vi "Read Calib File.vi"(8 "Inst type":T1=enum."Pressure Transducer", 11 "Calib File":path) -> (0 "Coefficients Found?":bool, 3 "Calib Constants":dbl[](array[numeric]))   [LabVIEW 2022 SP3]
uses:
  Controls/Inst_type.ctl
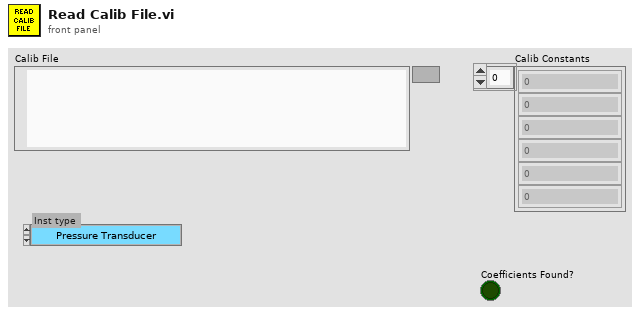
[diagram p1: front panel]
types:
  T1 = typedef "Inst_type.ctl" = enum16{"Raw voltage", "Raw with zero offsetting", "Propeller anemometer", "Pressure Transducer", "Pitot-static tube", "Hot wire", "Cross wire 1", "Cross wire 2", "Generic Linear", "Generic Polynomial", "Generic BackPoly", "Fast FID", "Thermocouple", "Cold wire", "Pulsed Wire", "LDA Vel", "LDA Tran time", "LDA Arr time", "Microphone"}
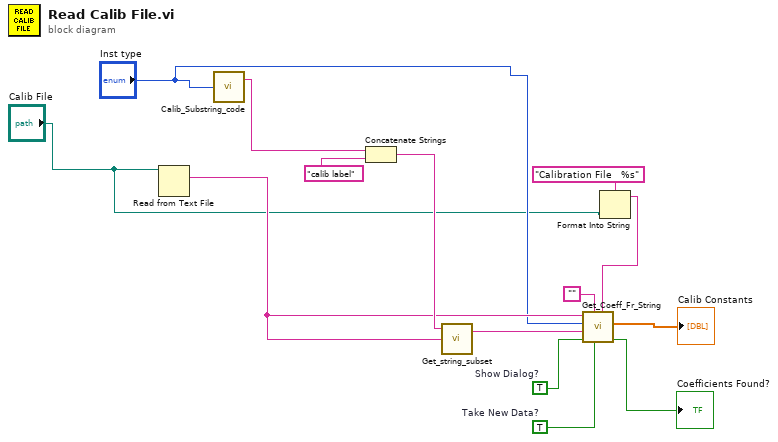
[diagram p0: block diagram]
diagram:
  w2 = TRUE  # Show Dialog?
  w3 = TRUE  # Take New Data?
  n1 = Read from Text File(file (use dialog)="Calib File") -> (text=w10:string)  [unwired: 3 in, 3 out]
  n2 = call "Calib_Substring_code.vi"("Inst type"="Inst type") -> ("Substring Type"=w13:string)  [unwired: 1 out]
  n3 = Concatenate Strings(w13, "calib label") -> (w12:string)
  n4 = call "Get_string_subset.vi"("String to split"=w10, "File Label"=w12) -> ("Output string"=w11:string)  [unwired: 2 in, 1 out]
  n5 = Format Into String(format string="Calibration File   %s", "Calib File") -> (resulting string=w5:string)  [unwired: 2 in, 1 out]
  n6 = call "Get_Coeff_Fr_String.vi"("String Name"=w5, "Take New Data?"=w3, "Prefix"="", "Show Dialog?"=w2, "Sub String"=w11, "Inst type"="Inst type", "Whole String"=w10) -> ("Coefficients Found?"=→"Coefficients Found?":bool, "Calib Constants"=→"Calib Constants":dbl[])  [unwired: 2 in]
